vi "Terminate.vi"(8 "error in (no error)":errorcluster, 10 "Message in":refnum<class "TerminateMessage.lvclass">, 11 "MeritFactor in":refnum<class "MeritFactor.lvclass">) -> (0 "error out":errorcluster, 3 "MeritFactor out":refnum<class "MeritFactor.lvclass">)   [LabVIEW 2012, in "MeritFactor.lvclass"]
doc: "This member function is called when the statemachine in the run.vi receives an 'terminate' command. It closes the RabbitMQ connection. \n\nOverride this member function in your derived class to release all previously acquired resources (but don't forget to call the parent method). If your component has subcomponents, they count as resources, and you have to release them by calling their own terminate functions."
uses:
  MeritFactor.lvclass
  <vilib>/Distrio/Murmex/TerminateMessage/TerminateMessage.lvclass
  MeritFactor.lvclass/MeritFactor.ctl
  <vilib>/Distrio/Murmex/Murmex/Murmex.lvclass
panel:
  # "This method is called when the TERMINATE\ntrigger is sent. \n\nOverride this method when your component needs to\nrespond to this trigger. \n\nCall parent for proper implementation"
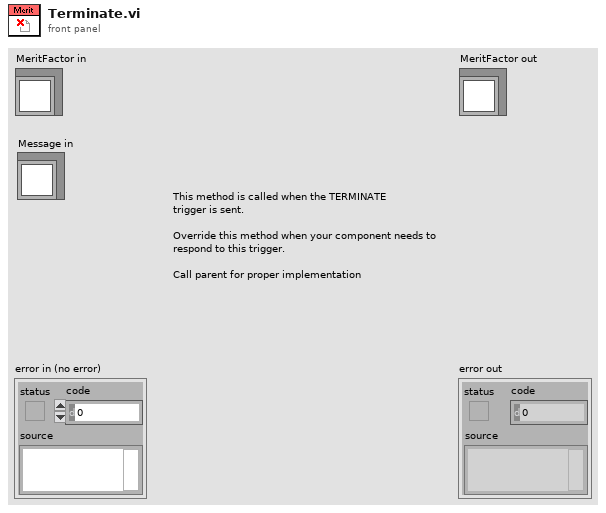
[diagram p1: front panel]
types:
  T1 = typedef "IMAQ Image.ctl" = refnum<image>
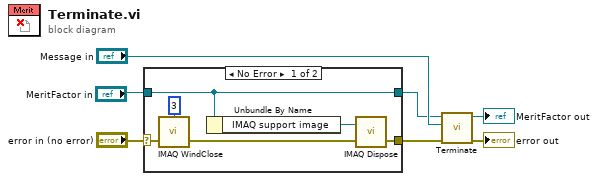
[diagram p0: block diagram]
diagram:
  n1 = case shown="No Error" "error in (no error)" {
    selector: "error in (no error)" -> [w13 w14]
    tunnel: [w10 w14] -> w4
    tunnel: "MeritFactor in" -> [w8 w15]
    tunnel: [w8 w15] -> w2
    frame No Error {
      n2 = call "IMAQ WindClose"("Window Number (0...15)"=3, "error in (no error)"=w13) -> ("error out"=w11:errorcluster)  [unwired: 4 in]
      n3 = Unbundle By Name(w8) -> ("IMAQ support image"=w9:T1)
      n4 = call "IMAQ Dispose"("Image"=w9, "error in (no error)"=w11) -> ("error out"=w10:errorcluster)  [unwired: 4 in]
    }
    frame Error {
    }
  }
  n5 = call-parent "Terminate.vi"("error in (no error)"=w4, "Message in"="Message in", "Murmex in"=w2) -> ("error out"=→"error out":errorcluster, "Murmex out"=→"MeritFactor out":refnum<class "MeritFactor.lvclass">)  [unwired: 7 in]
